vi "NISE.local.Get Command Documentation.vi"(0 "SLSC Local in":refnum<class "SLSC Interface.lvclass">, 5 "command":refnum<k21>, 11 "error in (no error)":errorcluster) -> (4 "SLSC Local out":refnum<class "SLSC Interface.lvclass">, 6 "command out":refnum<k21>, 10 "Cmd.Doc":string, 15 "error out":errorcluster)   [LabVIEW 2016, in "SLSC Interface.lvclass"]
uses:
  SLSC Interface Class/SLSC Interface.lvclass
  <resource>/objmgr/slsc.rc
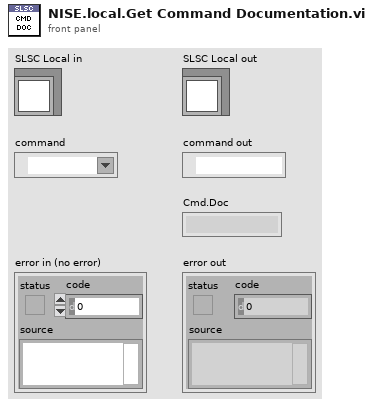
[diagram p1: front panel]
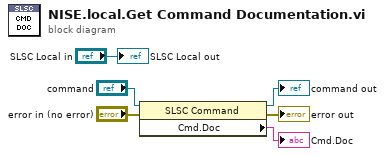
[diagram p0: block diagram]
diagram:
  n1 = property class="SLSC Command"(reference="command", error in="error in (no error)") -> (reference out=→"command out":refnum<k21>, error out=→"error out":errorcluster, "Cmd.Doc"=→"Cmd.Doc":string)
  "SLSC Local out" <- "SLSC Local in"
